vi "manejaBD.vi"(8 "error in":errorcluster, 10 "All Message Queues in":T1, 11 "Calibrador in":refnum<class "Calibrador.lvclass">) -> (0 "error out":errorcluster)   [LabVIEW 2019, in "Calibrador.lvclass"]
uses:
  Calibrador.lvclass
  QMH/Message Queue/All Message Queues.ctl
  QMH/Message Queue/Message Cluster.ctl
  Calibrador.lvclass/Calibrador.ctl
  <vilib>/Utility/error.llb/Error Cluster From Error Code.vi
  RerenceAllControlsToolkit/_get mutiple control reference by name.vi
  RerenceAllControlsToolkit/_get control reference by name.vi
  QMH/Message Queue/Enqueue Message (Single).vi
  <vilib>/ErrorRing/Error Ring.xnode
  Base de Datos/SQLiteConnector/SQLiteConnection.lvclass
  QMH/Message Queue/Message Queue.lvlib
  Base de Datos/Base de Datos.lvclass
  <vilib>/Utility/Data Type/NI_Data Type.lvlib
panel:
  out "All States":string[](array[string])
  out "Actual State":string
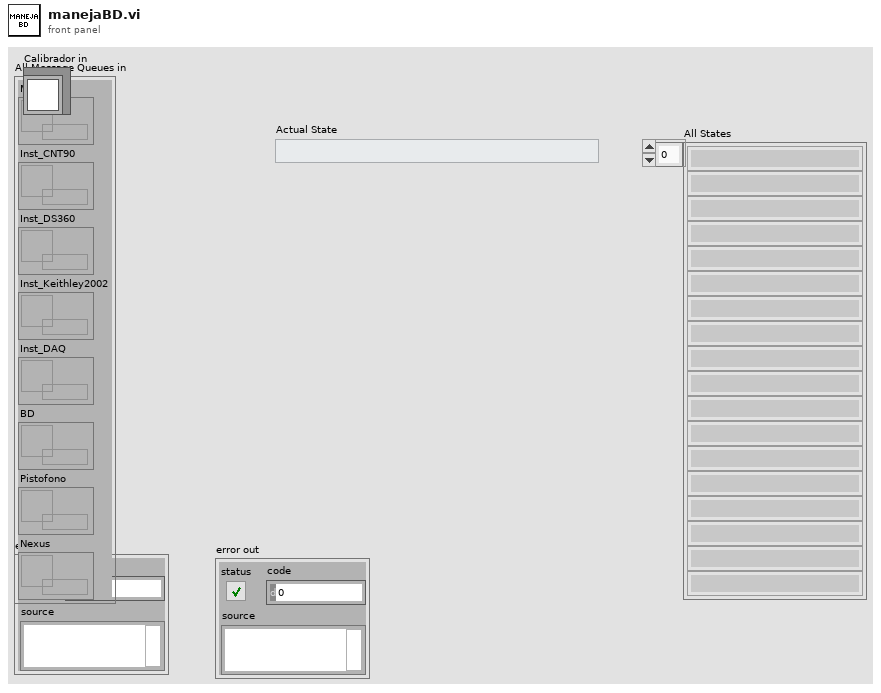
[diagram p1: front panel]
types:
  T1 = typedef "Message Queue.lvlib/All Message Queues.ctl" = cluster{"MHL":refnum<queue>, "Inst_CNT90":refnum<queue>, "Inst_DS360":refnum<queue>, "Inst_Keithley2002":refnum<queue>, "Inst_DAQ":refnum<queue>, "BD":refnum<queue>, "Pistofono":refnum<queue>, "Nexus":refnum<queue>}
  T2 = cluster{"Marca":string, "Referencia":cluster{"ControlName":string, "ControlReference":refnum<vi>}[]}
  T3 = typedef "NI_Data Type.lvlib/Data Type.ctl" = enum8{"Invalid Type", "Void", "I8", "I16", "I32", "I64", "U8", "U16", "U32", "U64", "Single Float", "Double Float", "Extended Float", "Single Complex", "Double Complex", "Extended Complex", "Enum U8", "Enum U16", "Enum U32", "Enum U64", "Single Float With Unit", "Double Float With Unit", "Extended Float With Unit", "Single Complex with Unit", "Double Complex with Unit", "Extended Complex with Unit", "Boolean", "String", "Path", "Picture", "Tag", "Array", "Cluster", "Variant", "LV Variant", "Waveform", "Timestamp", "Digital Waveform", "Digital Data", "ExpressData", "Refnum", "External Data", "VI", "Poly VI", "LabVIEW Class Instance", "Fixed Point", "Set Collection", "Map Collection"}
  T4 = cluster{"ControlName":string, "ControlReference":refnum<vi>}[]
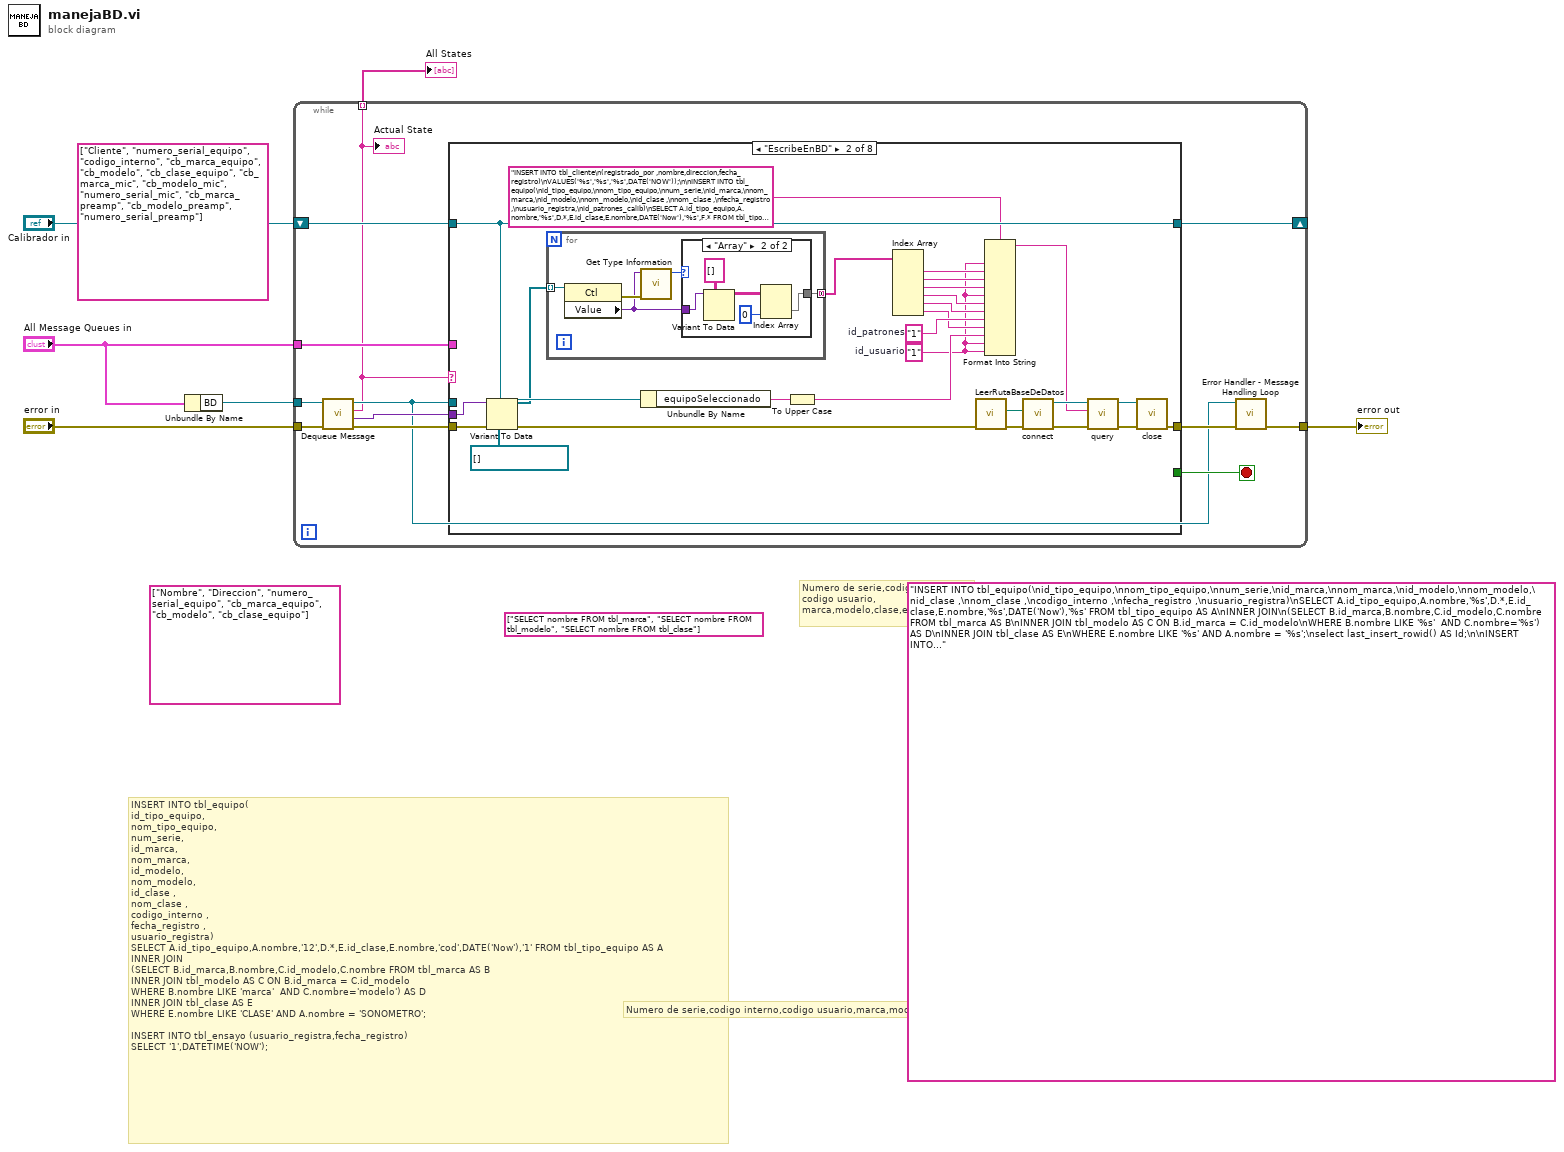
[diagram p0: block diagram]
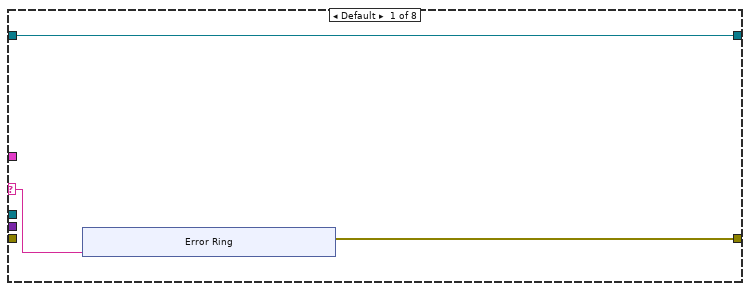
[diagram p2: hidden frame]
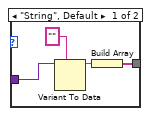
[diagram p3: hidden frame]
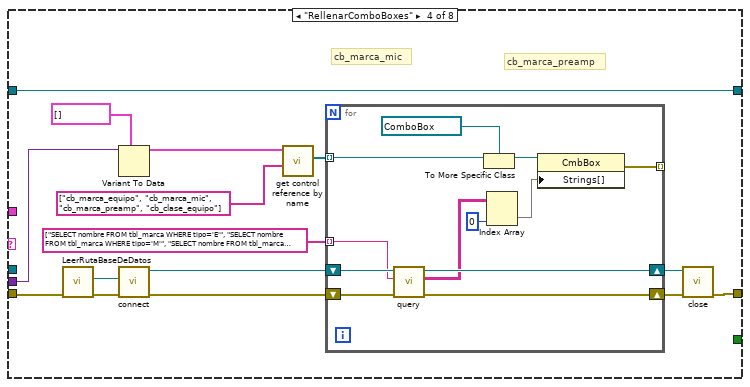
[diagram p5: hidden frame]
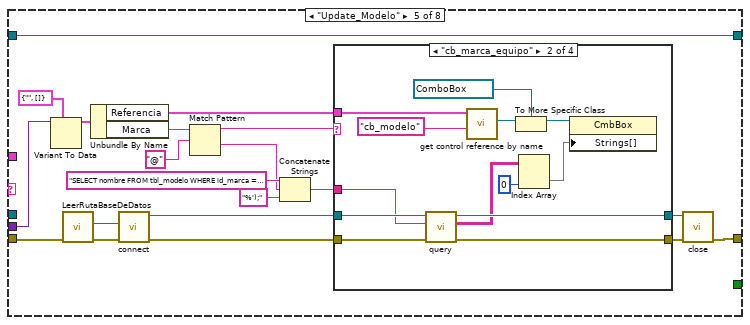
[diagram p6: hidden frame]
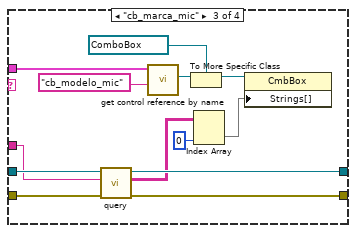
[diagram p8: hidden frame]
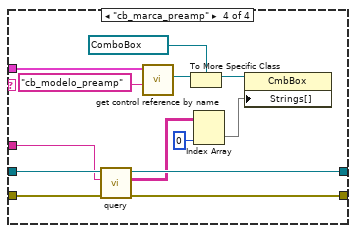
[diagram p9: hidden frame]
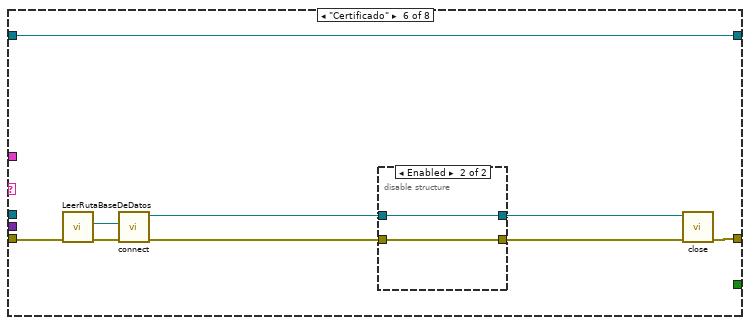
[diagram p10: hidden frame]
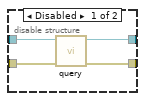
[diagram p11: hidden frame]
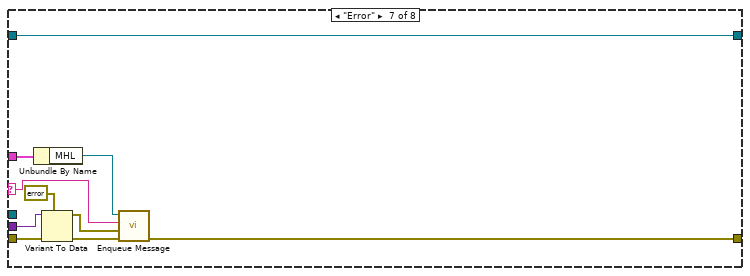
[diagram p12: hidden frame]
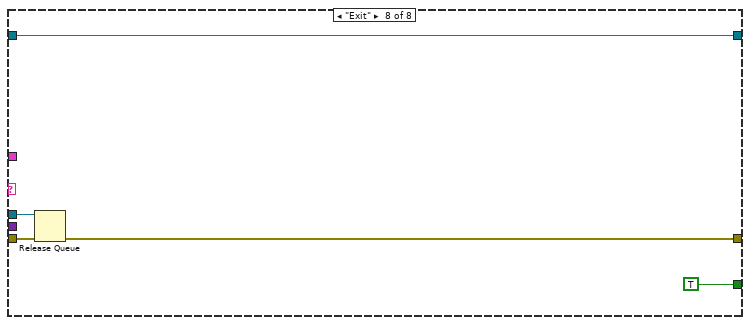
[diagram p13: hidden frame]
diagram:
  (unwired) string[] ["Cliente", "numero_serial_equipo", "codigo_interno", "cb_marca_equipo", "cb_modelo", "cb_clase_equipo", "cb_marca_mic", "cb_modelo_mic", "numero_serial_mic", "cb_marca_preamp", "cb_modelo_preamp", "numero_serial_preamp"]
  (unwired) string[] ["Nombre", "Direccion", "numero_serial_equipo", "cb_marca_equipo", "cb_modelo", "cb_clase_equipo"]
  (unwired) "INSERT INTO tbl_equipo(\nid_tipo_equipo,\nnom_tipo_equipo,\nnum_serie,\nid_marca,\nnom_marca,\nid_modelo,\nnom_modelo,\nid_clase ,\nnom_clase ,\ncodigo_interno ,\nfecha_registro ,\nusuario_registra)\nSELECT A.id_tipo_equipo,A.nombre,'%s',D.*,E.id_clase,E.nombre,'%s',DATE('Now'),'%s' FROM tbl_tipo_equipo AS A\nINNER JOIN\n(SELECT B.id_marca,B.nombre,C.id_modelo,C.nombre FROM tbl_marca AS B\nINNER JOIN tbl_modelo AS C ON B.id_marca = C.id_modelo\nWHERE B.nombre LIKE '%s'  AND C.nombre='%s') AS D\nINNER JOIN tbl_clase AS E\nWHERE E.nombre LIKE '%s' AND A.nombre = '%s';\nselect last_insert_rowid() AS Id;\n\nINSERT INTO tbl_info_ensayo (id_ensayo,id_equipo,id_cliente,id_cond_amb_iniciales,id_clase_pruebas)\nSELECT (SELECT MAX(id_ensayo) FROM tbl_ensayo) AS id_ensayo,(SELECT MAX(id_equipo) FROM tbl_equipo) AS id_equipo,'%s' AS id_cliente,(SELECT MAX(id_cond_amb_iniciales) FROM tbl_cond_amb_iniciales) AS id_cond_amb_iniciales,\n(SELECT id_clase_prueba FROM tbl_clase_prueba WHERE id_clase=(SELECT id_clase FROM tbl_equipo ORDER BY id_equipo DESC LIMIT 1)  AND id_prueba=(SELECT id_prueba FROM tbl_prueba Where nombre='%s')) AS id_clase_pruebas;\n"
  (unwired) string[] ["SELECT nombre FROM tbl_marca", "SELECT nombre FROM tbl_modelo", "SELECT nombre FROM tbl_clase"]
  # "INSERT INTO tbl_equipo(\nid_tipo_equipo,\nnom_tipo_equipo,\nnum_serie,\nid_marca,\nnom_marca,\nid_modelo,\nnom_modelo,\nid_clase ,\nnom_clase ,\ncodigo_interno ,\nfecha_registro ,\nusuario_registra)\nSELECT A.id_tipo_equipo,A.nombre,'12',D.*,E.id_clase,E.nombre,'cod',DATE('Now'),'1' FROM tbl_tipo_equipo AS A\nINNER JOIN\n(SELECT B.id_marca,B.nombre,C.id_modelo,C.nombre FROM tbl_marca AS B\nINNER JOIN tbl_modelo AS C ON B.id_marca = C.id_modelo\nWHERE B.nombre LIKE 'marca'  AND C.nombre='modelo') AS D\nINNER JOIN tbl_clase AS E\nWHERE E.nombre LIKE 'CLASE' AND A.nombre = 'SONOMETRO';\n\nINSERT INTO tbl_ensayo (usuario_registra,fecha_registro)\nSELECT '1',DATETIME('NOW');"
  # "Numero de serie,codigo interno,\ncodigo usuario,\nmarca,modelo,clase,equipo"
  # "Numero de serie,codigo interno,codigo usuario,marca,modelo,equipo,clase"
  # "BD Ref"
  n1 = Unbundle By Name("All Message Queues in") -> ("BD"=w4:refnum<queue>)
  n2 = while {
    tunnel: "error in" -> [w18]
    tunnel: w4 -> [w17]
    tunnel: "All Message Queues in" -> [w16]
    tunnel: [w9] -> w2
    shift-right: [w12] -> _
    shift-left: "Calibrador in" -> [w15]
    tunnel: [w7] -> w1 mode=indexing
    stop <- w11 stop-if-true
    n3 = call "Dequeue Message.vi"("error in (no error)"=w18, "Message Queue"=w17) -> ("error out"=w13:errorcluster, "Message Data"=w14:variant, "Message"=w7:string, "dup Message Queue"=w8:refnum<queue>)  [unwired: 6 in]
    "Actual State" <- w7
    n4 = case shown="\"EscribeEnBD\"" w7 {
      selector: w7 -> [w21 _ _ _ _ _ w178 _]
      tunnel: w16 -> [_ _ _ _ _ _ w177 _]
      tunnel: w15 -> [w19 w49 w70 w71 w117 w167 w175 w185]
      tunnel: w8 -> [_ _ _ _ _ _ _ w187]
      tunnel: w14 -> [_ w51 _ w78 w109 _ w181 _]
      tunnel: w13 -> [_ w53 w69 w81 w112 w162 w182 w188]
      tunnel: [w20 w54 w69 w79 w110 w160 w174 w184] -> w10
      tunnel: [w19 w49 w70 w71 w117 w167 w175 w185] -> w12
      tunnel: [_ _ _ _ _ _ _ TRUE] -> w11
      frame Default {
        n5 = xnode "Error Ring"("parameter 0"=w21) -> ("error out"=w20:errorcluster)
      }
      frame "EscribeEnBD" {
        w32 = "1"  # id_patrones
        w29 = "1"  # id_usuario
        n6 = Variant To Data(error in=w53, type=refnum<vi>[] [], Variant=w51) -> (data=w35:refnum<vi>[], error out=w52:errorcluster)
        n7 = for {
          tunnel: w35 -> [w59] mode=indexing
          tunnel: [w58] -> w34 mode=concatenating
          n8 = property class="Ctl"(reference=w59) -> (error out=w57:errorcluster, "Value"=w56:variant)  [unwired: 1 in, 1 out]
          n9 = call <vilib>:"Get Type Information.vi"("error in (no error)"=w57, "variant"=w56) -> ("type"=w55:T3)  [unwired: 5 in, 4 out]
          n10 = case shown="\"Array\"" w55 {
            tunnel: [w60 w65] -> w58
            tunnel: w56 -> [w62 w67]
            frame "String", Default {
              n11 = Variant To Data(type="", Variant=w62) -> (data=w61:string)  [unwired: 1 in, 1 out]
              n12 = Build Array(w61) -> (w60:string[])
            }
            frame "Array" {
              n13 = Variant To Data(type=string[][] [], Variant=w67) -> (data=w66:string[][])  [unwired: 1 in, 1 out]
              n14 = Index Array(array=w66, index (col)=0 ("disabled index (col)")) -> (element=w65:string[])  [unwired: 1 in]
            }
          }
        }
        n15 = Unbundle By Name(w49) -> ("equipoSeleccionado"=w36:string)
        n16 = To Upper Case(1:w36) -> (0:w30:string)
        n17 = Index Array(array=w34) -> (element #1=w33:string, element #2=w41:string, element #3=w40:string, element #4=w39:string, element #5=w38:string, element #6=w31:string)  [unwired: 6 in]
        n18 = call "LeerRutaBaseDeDatos.vi"("error in (no error)"=w52) -> ("error out"=w44:errorcluster, "Database Path"=w43:path)  [unwired: 9 in]
        n19 = Format Into String(format string="INSERT INTO tbl_cliente\n(registrado_por ,nombre,direccion,fecha_registro)\nVALUES('%s','%s','%s',DATE('NOW'));\n\nINSERT INTO tbl_equipo(\nid_tipo_equipo,\nnom_tipo_equipo,\nnum_serie,\nid_marca,\nnom_marca,\nid_modelo,\nnom_modelo,\nid_clase ,\nnom_clase ,\nfecha_registro ,\nusuario_registra,\nid_patrones_calib)\nSELECT A.id_tipo_equipo,A.nombre,'%s',D.*,E.id_clase,E.nombre,DATE('Now'),'%s',F.* FROM tbl_tipo_equipo AS A\nINNER JOIN\n(SELECT B.id_marca,B.nombre,C.id_modelo,C.nombre FROM tbl_marca AS B\nINNER JOIN tbl_modelo AS C ON B.id_marca = C.id_marca\nWHERE B.nombre LIKE '%s'  AND C.nombre='%s') AS D\nINNER JOIN tbl_clase AS E\nINNER JOIN (SELECT '%s') AS F\nWHERE E.nombre LIKE '%s' AND A.nombre = '%s';\n\nINSERT INTO tbl_equipo_cliente(id_cliente,nom_cliente,id_equipo,fecha_registro,usuario_registra)\nSELECT MAX(id_cliente),nombre,last_insert_rowid(),DATETIME('NOW'),'%s' FROM tbl_cliente;\n\nINSERT INTO tbl_ensayo (usuario_registra,fecha_registro)\nSELECT '%s',DATETIME('NOW');", w29, w33, w41, w40, w29, w39, w38, w32, w31, w30, w29, w29) -> (resulting string=w37:string)  [unwired: 2 in, 1 out]
        n20 = call "connect.vi"("error in (no error)"=w44, "Database Path"=w43) -> ("error out"=w46:errorcluster, "object out"=w45:refnum<class "SQLiteConnection.lvclass">)  [unwired: 8 in]
        n21 = call "query.vi"("error in (no error)"=w46, "SQL Statement"=w37, "object in"=w45) -> ("error out"=w48:errorcluster, "object out"=w47:refnum<class "SQLiteConnection.lvclass">)  [unwired: 5 in, 2 out]
        n22 = call-dynamic "close.vi"("error in (no error)"=w48, "object in"=w47) -> ("error out"=w54:errorcluster)  [unwired: 8 in, 1 out]
      }
      frame "Initialize" {
      }
      frame "RellenarComboBoxes" {
        # "cb_marca_preamp"
        # "cb_marca_mic"
        n23 = call "LeerRutaBaseDeDatos.vi"("error in (no error)"=w81) -> ("error out"=w83:errorcluster, "Database Path"=w82:path)  [unwired: 9 in]
        n24 = Variant To Data(type=cluster{string, refnum<vi>}[] [] ("Control references"), Variant=w78) -> (data=w76:cluster{string, refnum<vi>}[])  [unwired: 1 in, 1 out]
        n25 = call "connect.vi"("error in (no error)"=w83, "Database Path"=w82) -> ("error out"=w84:errorcluster, "object out"=w85:refnum<class "SQLiteConnection.lvclass">)  [unwired: 8 in]
        n26 = call-poly "get control reference by name.vi"("Control names"=string[] ["cb_marca_equipo", "cb_marca_mic", "cb_marca_preamp", "cb_clase_equipo"] ("Control name"), "Control references"=w76) -> ("References"=w74:refnum<vi>[])  [unwired: 4 in, 1 out]
        n27 = for {
          tunnel: w74 -> [w92] mode=indexing
          shift-right: [w95] -> w80
          shift-left: w85 -> [w97]
          shift-right: [w88] -> w73
          shift-left: w84 -> [w96]
          tunnel: string[] ["SELECT nombre FROM tbl_marca WHERE tipo='E'", "SELECT nombre FROM tbl_marca WHERE tipo='M'", "SELECT nombre FROM tbl_marca WHERE tipo='P'", "SELECT nombre FROM tbl_clase"] -> [w87] mode=indexing
          tunnel: [w86] -> _ mode=indexing
          n28 = call "query.vi"("error in (no error)"=w96, "SQL Statement"=w87, "object in"=w97) -> ("error out"=w88:errorcluster, "result"=w94:string[][], "object out"=w95:refnum<class "SQLiteConnection.lvclass">)  [unwired: 5 in, 1 out]
          n29 = To More Specific Class(target class=refnum<vi> refnum ("cb_marca_equipo"), reference=w92) -> (specific class reference=w91:refnum<vi>)  [unwired: 1 in, 1 out]
          n30 = Index Array(array=w94, index (col)=0 ("disabled index (col)")) -> (element=w89:string[])  [unwired: 1 in]
          n31 = property class="CmbBox"(reference=w91, "Strings[]"=w89) -> (error out=w86:errorcluster)  [unwired: 1 in, 1 out]
        }
        n32 = call-dynamic "close.vi"("error in (no error)"=w73, "object in"=w80) -> ("error out"=w79:errorcluster)  [unwired: 8 in, 1 out]
      }
      frame "Update_Modelo" {
        n33 = Variant To Data(type=T2 {"Marca"="", "Referencia"=[]} ("output cluster"), Variant=w109) -> (data=w106:T2)  [unwired: 1 in, 1 out]
        n34 = call "LeerRutaBaseDeDatos.vi"("error in (no error)"=w112) -> ("error out"=w114:errorcluster, "Database Path"=w113:path)  [unwired: 9 in]
        n35 = Unbundle By Name(w106) -> ("Referencia"=w105:T4, "Marca"=w103:string)
        n36 = call "connect.vi"("error in (no error)"=w114, "Database Path"=w113) -> ("error out"=w115:errorcluster, "object out"=w116:refnum<class "SQLiteConnection.lvclass">)  [unwired: 8 in]
        n37 = Match Pattern(string=w103, regular expression="@") -> (before substring=w104:string, after substring=w100:string)  [unwired: 1 in, 2 out]
        n38 = Concatenate Strings("SELECT nombre FROM tbl_modelo WHERE id_marca = (SELECT id_marca FROM tbl_marca WHERE nombre LIKE '%" ("SQL Statement"), w100, "%');" ("string")) -> (w98:string)
        n39 = case shown="\"cb_marca_equipo\"" w104 {
          tunnel: w116 -> [w119 w132 w145 w158]
          tunnel: w115 -> [w118 w131 w144 w157]
          tunnel: [w119 w130 w143 w156] -> w111
          tunnel: [w118 w128 w141 w154] -> w108
          tunnel: w105 -> [_ w121 w134 w147]
          tunnel: w98 -> [_ w120 w133 w146]
          frame "False", Default {
          }
          frame "cb_marca_equipo" {
            n40 = call "query.vi"("error in (no error)"=w131, "SQL Statement"=w120, "object in"=w132) -> ("error out"=w128:errorcluster, "result"=w127:string[][], "object out"=w130:refnum<class "SQLiteConnection.lvclass">)  [unwired: 5 in, 1 out]
            n41 = call-poly "get control reference by name.vi"("Control name"="cb_modelo", "Control references"=w121) -> ("Ctl Refnum"=w129:refnum<vi>)  [unwired: 4 in, 1 out]
            n42 = To More Specific Class(target class=refnum<vi> refnum ("cb_marca_equipo"), reference=w129) -> (specific class reference=w125:refnum<vi>)  [unwired: 1 in, 1 out]
            n43 = Index Array(array=w127, index (col)=0 ("disabled index (col)")) -> (element=w123:string[])  [unwired: 1 in]
            n44 = property class="CmbBox"(reference=w125, "Strings[]"=w123) -> ()  [unwired: 1 in, 2 out]
          }
          frame "cb_marca_mic" {
            n45 = call "query.vi"("error in (no error)"=w144, "SQL Statement"=w133, "object in"=w145) -> ("error out"=w141:errorcluster, "result"=w140:string[][], "object out"=w143:refnum<class "SQLiteConnection.lvclass">)  [unwired: 5 in, 1 out]
            n46 = call-poly "get control reference by name.vi"("Control name"="cb_modelo_mic", "Control references"=w134) -> ("Ctl Refnum"=w142:refnum<vi>)  [unwired: 4 in, 1 out]
            n47 = To More Specific Class(target class=refnum<vi> refnum ("cb_marca_equipo"), reference=w142) -> (specific class reference=w138:refnum<vi>)  [unwired: 1 in, 1 out]
            n48 = Index Array(array=w140, index (col)=0 ("disabled index (col)")) -> (element=w136:string[])  [unwired: 1 in]
            n49 = property class="CmbBox"(reference=w138, "Strings[]"=w136) -> ()  [unwired: 1 in, 2 out]
          }
          frame "cb_marca_preamp" {
            n50 = call "query.vi"("error in (no error)"=w157, "SQL Statement"=w146, "object in"=w158) -> ("error out"=w154:errorcluster, "result"=w153:string[][], "object out"=w156:refnum<class "SQLiteConnection.lvclass">)  [unwired: 5 in, 1 out]
            n51 = call-poly "get control reference by name.vi"("Control name"="cb_modelo_preamp", "Control references"=w147) -> ("Ctl Refnum"=w155:refnum<vi>)  [unwired: 4 in, 1 out]
            n52 = To More Specific Class(target class=refnum<vi> refnum ("cb_marca_equipo"), reference=w155) -> (specific class reference=w151:refnum<vi>)  [unwired: 1 in, 1 out]
            n53 = Index Array(array=w153, index (col)=0 ("disabled index (col)")) -> (element=w149:string[])  [unwired: 1 in]
            n54 = property class="CmbBox"(reference=w151, "Strings[]"=w149) -> ()  [unwired: 1 in, 2 out]
          }
        }
        n55 = call-dynamic "close.vi"("error in (no error)"=w108, "object in"=w111) -> ("error out"=w110:errorcluster)  [unwired: 8 in, 1 out]
      }
      frame "Certificado" {
        n56 = call "LeerRutaBaseDeDatos.vi"("error in (no error)"=w162) -> ("error out"=w164:errorcluster, "Database Path"=w163:path)  [unwired: 9 in]
        n57 = call "connect.vi"("error in (no error)"=w164, "Database Path"=w163) -> ("error out"=w165:errorcluster, "object out"=w166:refnum<class "SQLiteConnection.lvclass">)  [unwired: 8 in]
        n58 = disable-structure shown="Enabled" {
          disable-tunnel: w166 -> [w171 w173]
          disable-tunnel: w165 -> [w170 w172]
          disable-tunnel: [w169 w173] -> w161
          disable-tunnel: [w168 w172] -> w159
          frame Disabled {
            n59 = call "query.vi"("error in (no error)"=w170, "object in"=w171) -> ("error out"=w168:errorcluster, "object out"=w169:refnum<class "SQLiteConnection.lvclass">)  [unwired: 6 in, 2 out]
          }
          frame Enabled {
          }
        }
        n60 = call-dynamic "close.vi"("error in (no error)"=w159, "object in"=w161) -> ("error out"=w160:errorcluster)  [unwired: 8 in, 1 out]
      }
      frame "Error" {
        n61 = Unbundle By Name(w177) -> ("MHL"=w176:refnum<queue>)
        n62 = Variant To Data(error in=w182, type=errorcluster {"status"=FALSE, "code"=0, "source"=""} ("error constant"), Variant=w181) -> (data=w179:errorcluster, error out=w180:errorcluster)
        n63 = call-poly "Enqueue Message.vi"("error in (no error)"=w180, "Message Data"=w179, "Message"=w178, "Message Queue"=w176) -> ("error out"=w174:errorcluster)  [unwired: 6 in, 1 out]
      }
      frame "Exit" {
        n64 = Release Queue(queue=w187, error in (no error)=w188) -> (error out=w184:errorcluster)  [unwired: 1 in, 2 out]
      }
    }
    n65 = call "Error Handler - Message Handling Loop.vi"("error in (no error)"=w10, "Message Queue"=w8) -> ("dup error in"=w9:errorcluster)  [unwired: 8 in, 1 out]
  }
  "error out" <- w2
  "All States" <- w1
